vi "Partition_Setup.vi"(8 "error in (no error)":errorcluster, 11 "DataCluster in":T1={"Core"={"Current VI Reference"=refnum, "Close Panel on Exit?"=FALSE, "Exit"=FALSE, "Initialized?"=FALSE}, "Connections"={"cDAQ"={"Task"="ThermTask", "Connected"=FALSE, "Active"=FALSE, "ID"=""}, "Camera"={"Session"="", "Connected"=FALSE, "Active"=FALSE, "Placeholder"=refnum}, "PSU"={"Port"="", "Connected"=FALSE, "Active"=FALSE}, "Arduino"={"Port"="", "Connected"=FALSE, "Active"=FALSE}}, "Data Acquisition"={"Setup"={"Label"="_41", "Operator"="", "Notes"="", "TempGrad"=1.0, "TargetTemp"=-20.0, "Sample Volume"=1.0}, "Camera"={"Image"=refnum, "Save Image"=refnum, "Image Frequency"=20, "Rectangle"={"Left"=0, "Top"=0, "Right"=0, "Bottom"=0, "Rotation"=0.0}, "Calibration"={"Top Left"={"X"=0.0, "Y"=0.0}, "Top Right"={"X"=0.0, "Y"=0.0}, "Bottom Left"={"X"=0.0, "Y"=0.0}, "Bottom Right"={"X"=0.0, "Y"=0.0}, "Fixpoint"={"X"=0.0, "Y"=0.0}, "Scan Area"=0.0, "Fixpoint Area"=0.0, "Well Pixels"=[], "Valid"=FALSE}, "FocusPos"=0, "Display Mapping"=10, "Camera Mode"=10}, "Thermistor"={"Sample Size"=5, "Calibration"={"B0.100"=[3450.0, 3450.0, 3450.0, 3450.0, 3450.0, 3450.0, 3450.0, 3450.0], "R25"=[10.74, 10.74, 10.74, 10.74, 10.74, 10.74, 10.74, 10.74], "c"=[], "State"=[], "V_S"=10.0, "R_S"=10.0}, "Timing Mode"=14713}, "Partition"={"Data"=[], "Cell Label"="", "Cell Color"=0, "Height"=10, "Width"=16, "Grid"=[]}, "Queue"={"Size"=5, "Queue"=refnum}, "Sample Rate"=240, "Active"=FALSE, "Ready"=FALSE, "Graph Mode"=0, "Gradient Buffer"=2}, "Control"={"Sample Rate"=20, "PID gains"={"proportional gain (Kc)"=1.0, "integral time (Ti, min)"=0.01, "derivative time (Td, min)"=0.0}}, "Manual Temp Control"={"TargetTemp"=1.0, "Mode"=0, "Active"=FALSE}} {"Manual Temp Control"."Mode" items=["Cool", "Heat"]; "Manual Temp Control"."TargetTemp" min=-40.0 max=40.0 step=0.5 format="%#_g °C"; "Control"."PID gains"."derivative time (Td, min)" format="%.3f"; "Control"."PID gains"."integral time (Ti, min)" format="%.3f"; "Control"."PID gains"."proportional gain (Kc)" format="%.3f"; "Control"."Sample Rate" min=1 max=20 step=1 format="%.0f Samples/sec"; "Data Acquisition"."Gradient Buffer" min=2 max=30 step=1; "Data Acquisition"."Graph Mode" items=["Thermistor Temperature", "Camera Temperature"]; "Data Acquisition"."Thermistor"."Timing Mode" items=["Automatic"=16097, "High Resolution"=10195, "High Speed"=14712, "Best 50 Hz Rejection"=14713, "Best 60 Hz Rejection"=14714, "Custom"=10137]; "Data Acquisition"."Thermistor"."Calibration"."R_S" min=0.1 max=1000.0 format="%#_g kOhm"; "Data Acquisition"."Thermistor"."Calibration"."V_S" min=5.0 max=48.0 format="%#_g V"; "Data Acquisition"."Thermistor"."Calibration"."R25" min=0.1 max=1000.0 format="%#_g kOhm"; "Data Acquisition"."Thermistor"."Calibration"."B0.100" min=100.0 max=10000.0 format="%#_g K"; "Data Acquisition"."Thermistor"."Sample Size" min=1 max=200; "Data Acquisition"."Sample Rate" min=20 max=240 format="%.0f samples/min"; "Data Acquisition"."Queue"."Size" min=1 max=200; "Data Acquisition"."Camera"."Camera Mode" items=["Temperature Linear", "Signal Linear"]; "Data Acquisition"."Camera"."Display Mapping" items=["Default"=10, "Most Significant Bits"=11, "Full Dynamic"=12, "Downshift"=13, "Given Range"=14, "90% Dynamic"=15, "Given Percent Range"=16]; "Data Acquisition"."Camera"."Calibration"."Fixpoint"."Y" format="%.2f"; "Data Acquisition"."Camera"."Calibration"."Fixpoint"."X" format="%.2f"; "Data Acquisition"."Camera"."Calibration"."Top Left"."Y" format="%.2f"; "Data Acquisition"."Camera"."Calibration"."Top Left"."X" format="%.2f"; "Data Acquisition"."Camera"."Calibration"."Top Right"."Y" format="%.2f"; "Data Acquisition"."Camera"."Calibration"."Top Right"."X" format="%.2f"; "Data Acquisition"."Camera"."Calibration"."Bottom Left"."Y" format="%.2f"; "Data Acquisition"."Camera"."Calibration"."Bottom Left"."X" format="%.2f"; "Data Acquisition"."Camera"."Calibration"."Bottom Right"."Y" format="%.2f"; "Data Acquisition"."Camera"."Calibration"."Bottom Right"."X" format="%.2f"; "Data Acquisition"."Camera"."Rectangle"."Rotation" min=-90.0 max=90.0 step=1.0 format="%.2f"; "Data Acquisition"."Camera"."Rectangle"."Left" scale=0.0..1024.0; "Data Acquisition"."Camera"."Rectangle"."Right" scale=0.0..1024.0; "Data Acquisition"."Camera"."Image Frequency" min=1 max=60 step=1; "Data Acquisition"."Setup"."Sample Volume" min=0.0 max=500.0 format="%#_g µL"; "Data Acquisition"."Setup"."TargetTemp" min=-40.0 max=40.0 step=0.5 format="%#_g °C"; "Data Acquisition"."Setup"."TempGrad" min=-100.0 max=100.0 step=0.1 format="%#_g °C/min"}) -> (0 "error out":errorcluster, 2 "Canceled?":bool, 3 "DataCluster out":T1={"Core"={"Current VI Reference"=refnum, "Close Panel on Exit?"=FALSE, "Exit"=FALSE, "Initialized?"=FALSE}, "Connections"={"cDAQ"={"Task"="ThermTask", "Connected"=FALSE, "Active"=FALSE, "ID"=""}, "Camera"={"Session"="", "Connected"=FALSE, "Active"=FALSE, "Placeholder"=refnum}, "PSU"={"Port"="", "Connected"=FALSE, "Active"=FALSE}, "Arduino"={"Port"="", "Connected"=FALSE, "Active"=FALSE}}, "Data Acquisition"={"Setup"={"Label"="_41", "Operator"="", "Notes"="", "TempGrad"=1.0, "TargetTemp"=-20.0, "Sample Volume"=1.0}, "Camera"={"Image"=refnum, "Save Image"=refnum, "Image Frequency"=20, "Rectangle"={"Left"=0, "Top"=0, "Right"=0, "Bottom"=0, "Rotation"=0.0}, "Calibration"={"Top Left"={"X"=0.0, "Y"=0.0}, "Top Right"={"X"=0.0, "Y"=0.0}, "Bottom Left"={"X"=0.0, "Y"=0.0}, "Bottom Right"={"X"=0.0, "Y"=0.0}, "Fixpoint"={"X"=0.0, "Y"=0.0}, "Scan Area"=0.0, "Fixpoint Area"=0.0, "Well Pixels"=[], "Valid"=FALSE}, "FocusPos"=0, "Display Mapping"=10, "Camera Mode"=10}, "Thermistor"={"Sample Size"=5, "Calibration"={"B0.100"=[3450.0, 3450.0, 3450.0, 3450.0, 3450.0, 3450.0, 3450.0, 3450.0], "R25"=[10.74, 10.74, 10.74, 10.74, 10.74, 10.74, 10.74, 10.74], "c"=[], "State"=[], "V_S"=10.0, "R_S"=10.0}, "Timing Mode"=14713}, "Partition"={"Data"=[["A", "20%", "", "", ""], ["B", "30", "", "", ""], ["C", "5%", "", "", ""], ["D", "35%", "", "", ""], ["E", "...", "", "", ""], ["F", "...", "", "", ""], ["G", "...", "", "", ""], ["X", "Empty", "", "", ""]], "Cell Label"="A", "Cell Color"=29373, "Height"=8, "Width"=12, "Grid"=[["X", "X", "X", "X", "X", "X", "X", "X", "X", "X", "X", "X"], ["X", "X", "X", "X", "X", "X", "X", "X", "X", "X", "X", "X"], ["X", "X", "X", "X", "X", "X", "X", "X", "X", "X", "X", "X"], ["X", "X", "X", "X", "X", "X", "X", "X", "X", "X", "X", "X"], ["X", "X", "X", "X", "X", "X", "X", "X", "X", "X", "X", "X"], ["X", "X", "X", "X", "X", "X", "X", "X", "X", "X", "X", "X"], ["X", "X", "X", "X", "X", "X", "X", "X", "X", "X", "X", "X"], ["X", "X", "X", "X", "X", "X", "X", "X", "X", "X", "X", "X"]]}, "Queue"={"Size"=5, "Queue"=refnum}, "Sample Rate"=240, "Active"=FALSE, "Ready"=FALSE, "Graph Mode"=0, "Gradient Buffer"=2}, "Control"={"Sample Rate"=20, "PID gains"={"proportional gain (Kc)"=1.0, "integral time (Ti, min)"=0.01, "derivative time (Td, min)"=0.0}}, "Manual Temp Control"={"TargetTemp"=1.0, "Mode"=0, "Active"=FALSE}} {"Manual Temp Control"."Mode" items=["Cool", "Heat"]; "Manual Temp Control"."TargetTemp" min=-40.0 max=40.0 step=0.5 format="%#_g °C"; "Control"."PID gains"."derivative time (Td, min)" format="%.3f"; "Control"."PID gains"."integral time (Ti, min)" format="%.3f"; "Control"."PID gains"."proportional gain (Kc)" format="%.3f"; "Control"."Sample Rate" min=1 max=20 step=1 format="%.0f Samples/sec"; "Data Acquisition"."Gradient Buffer" min=2 max=30 step=1; "Data Acquisition"."Graph Mode" items=["Thermistor Temperature", "Camera Temperature"]; "Data Acquisition"."Thermistor"."Timing Mode" items=["Automatic"=16097, "High Resolution"=10195, "High Speed"=14712, "Best 50 Hz Rejection"=14713, "Best 60 Hz Rejection"=14714, "Custom"=10137]; "Data Acquisition"."Thermistor"."Calibration"."R_S" min=0.1 max=1000.0 format="%#_g kOhm"; "Data Acquisition"."Thermistor"."Calibration"."V_S" min=5.0 max=48.0 format="%#_g V"; "Data Acquisition"."Thermistor"."Calibration"."R25" min=0.1 max=1000.0 format="%#_g kOhm"; "Data Acquisition"."Thermistor"."Calibration"."B0.100" min=100.0 max=10000.0 format="%#_g K"; "Data Acquisition"."Thermistor"."Sample Size" min=1 max=200; "Data Acquisition"."Sample Rate" min=20 max=240 format="%.0f samples/min"; "Data Acquisition"."Queue"."Size" min=1 max=200; "Data Acquisition"."Camera"."Camera Mode" items=["Temperature Linear", "Signal Linear"]; "Data Acquisition"."Camera"."Display Mapping" items=["Default"=10, "Most Significant Bits"=11, "Full Dynamic"=12, "Downshift"=13, "Given Range"=14, "90% Dynamic"=15, "Given Percent Range"=16]; "Data Acquisition"."Camera"."Calibration"."Fixpoint"."Y" format="%.2f"; "Data Acquisition"."Camera"."Calibration"."Fixpoint"."X" format="%.2f"; "Data Acquisition"."Camera"."Calibration"."Top Left"."Y" format="%.2f"; "Data Acquisition"."Camera"."Calibration"."Top Left"."X" format="%.2f"; "Data Acquisition"."Camera"."Calibration"."Top Right"."Y" format="%.2f"; "Data Acquisition"."Camera"."Calibration"."Top Right"."X" format="%.2f"; "Data Acquisition"."Camera"."Calibration"."Bottom Left"."Y" format="%.2f"; "Data Acquisition"."Camera"."Calibration"."Bottom Left"."X" format="%.2f"; "Data Acquisition"."Camera"."Calibration"."Bottom Right"."Y" format="%.2f"; "Data Acquisition"."Camera"."Calibration"."Bottom Right"."X" format="%.2f"; "Data Acquisition"."Camera"."Rectangle"."Rotation" min=-90.0 max=90.0 step=1.0 format="%.2f"; "Data Acquisition"."Camera"."Rectangle"."Left" scale=0.0..1024.0; "Data Acquisition"."Camera"."Rectangle"."Right" scale=0.0..1024.0; "Data Acquisition"."Camera"."Image Frequency" min=1 max=60 step=1; "Data Acquisition"."Setup"."Sample Volume" min=0.0 max=500.0 format="%#_g µL"; "Data Acquisition"."Setup"."TargetTemp" min=-40.0 max=40.0 step=0.5 format="%#_g °C"; "Data Acquisition"."Setup"."TempGrad" min=-100.0 max=100.0 step=0.1 format="%#_g °C/min"})   [LabVIEW 2024]
uses:
  DataCluster.ctl
  <vilib>/userDefined/High Color/IMAQdx.ctl
  <vilib>/vision/Image Controls.llb/IMAQ Image.ctl
  <vilib>/Utility/miscctls.llb/LVRowAndColumnTypeDef.ctl
  <vilib>/Utility/miscctls.llb/LVBoundsTypeDef.ctl
  <vilib>/Utility/xml.llb/Write to XML File(string).vi
  <vilib>/Utility/xml.llb/Read From XML File(string).vi
panel:
  out "Grid":string[][](table)=[["X", "X", "X", "X", "X", "X", "X", "X", "X", "X", "X", "X"], ["X", "X", "X", "X", "X", "X", "X", "X", "X", "X", "X", "X"], ["X", "X", "X", "X", "X", "X", "X", "X", "X", "X", "X", "X"], ["X", "X", "X", "X", "X", "X", "X", "X", "X", "X", "X", "X"], ["X", "X", "X", "X", "X", "X", "X", "X", "X", "X", "X", "X"], ["X", "X", "X", "X", "X", "X", "X", "X", "X", "X", "X", "X"], ["X", "X", "X", "X", "X", "X", "X", "X", "X", "X", "X", "X"], ["X", "X", "X", "X", "X", "X", "X", "X", "X", "X", "X", "X"]]
  in  "Cancel":bool
  in  "OK":bool
  in  "Partition Size":enum32{"12x8", "24x16"}(radio)
  in  "Partitions":i32[](listbox)=[0]
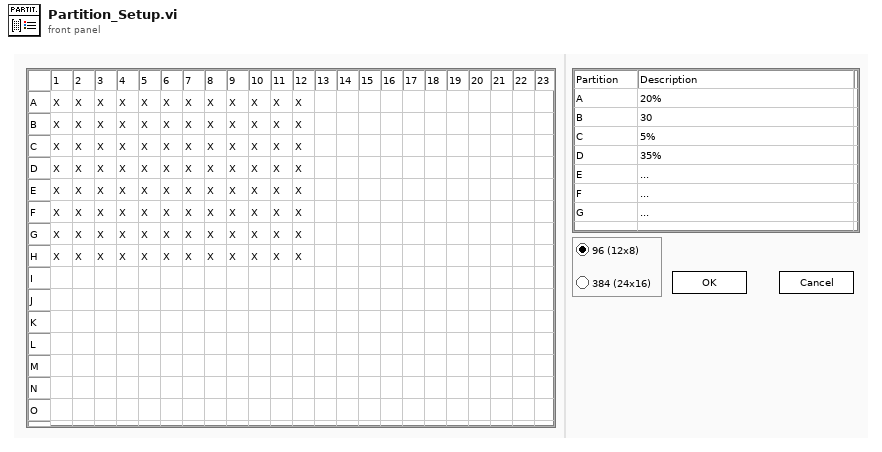
[diagram p1: front panel]
types:
  T1 = typedef "DataCluster.ctl" = cluster{"Core":cluster{"Current VI Reference":refnum<vi>, "Close Panel on Exit?":bool, "Exit":bool, "Initialized?":bool}, "Connections":cluster{"cDAQ":cluster{"Task":refnum<k21>, "Connected":bool, "Active":bool, "ID":string}, "Camera":cluster{"Session":T2, "Connected":bool, "Active":bool, "Placeholder":T3}, "PSU":cluster{"Port":refnum<visa-resource-name>, "Connected":bool, "Active":bool}, "Arduino":cluster{"Port":refnum<visa-resource-name>, "Connected":bool, "Active":bool}}, "Data Acquisition":cluster{"Setup":cluster{"Label":string, "Operator":string, "Notes":string, "TempGrad":dbl, "TargetTemp":dbl, "Sample Volume":dbl}, "Camera":cluster{"Image":T3, "Save Image":T3, "Image Frequency":i32, "Rectangle":T4, "Calibration":cluster{"Top Left":T5, "Top Right":T5, "Bottom Left":T5, "Bottom Right":T5, "Fixpoint":T5, "Scan Area":dbl, "Fixpoint Area":dbl, "Well Pixels":cluster{"X":i32, "Y":i32}[][], "Valid":bool}, "FocusPos":u32, "Display Mapping":u32, "Camera Mode":u32}, "Thermistor":cluster{"Sample Size":i32, "Calibration":cluster{"B0.100":dbl[], "R25":dbl[], "c":dbl[][], "State":bool[], "V_S":dbl, "R_S":dbl}, "Timing Mode":i32}, "Partition":cluster{"Data":string[][], "Cell Label":string, "Cell Color":u32, "Height":i32, "Width":i32, "Grid":string[][]}, "Queue":cluster{"Size":i32, "Queue":refnum<queue>}, "Sample Rate":i32, "Active":bool, "Ready":bool, "Graph Mode":u16, "Gradient Buffer":i32}, "Control":cluster{"Sample Rate":i32, "PID gains":cluster{"proportional gain (Kc)":dbl, "integral time (Ti, min)":dbl, "derivative time (Td, min)":dbl}}, "Manual Temp Control":cluster{"TargetTemp":dbl, "Mode":u16, "Active":bool}}
  T2 = typedef "IMAQdx.ctl" = refnum<k21>
  T3 = typedef "IMAQ Image.ctl" = refnum<image>
  T4 = typedef "IMAQ Rectangle" = cluster{"Left":i32, "Top":i32, "Right":i32, "Bottom":i32, "Rotation":dbl}
  T5 = typedef "IMAQ Point" = cluster{"X":sgl, "Y":sgl}
  T6 = typedef "LVRowAndColumnTypeDef.ctl" = cluster{"Row":i32, "Column":i32}
  T7 = cluster{"Data":string[][], "Cell Label":string, "Cell Color":u32, "Height":i32, "Width":i32, "Grid":string[][]}
  T8 = typedef "LVBoundsTypeDef.ctl" = cluster{"Width":u32, "Height":u32}
  T9 = typedef "LVRectTypeDef.ctl" = cluster{"Left":i16, "Top":i16, "Right":i16, "Bottom":i16}
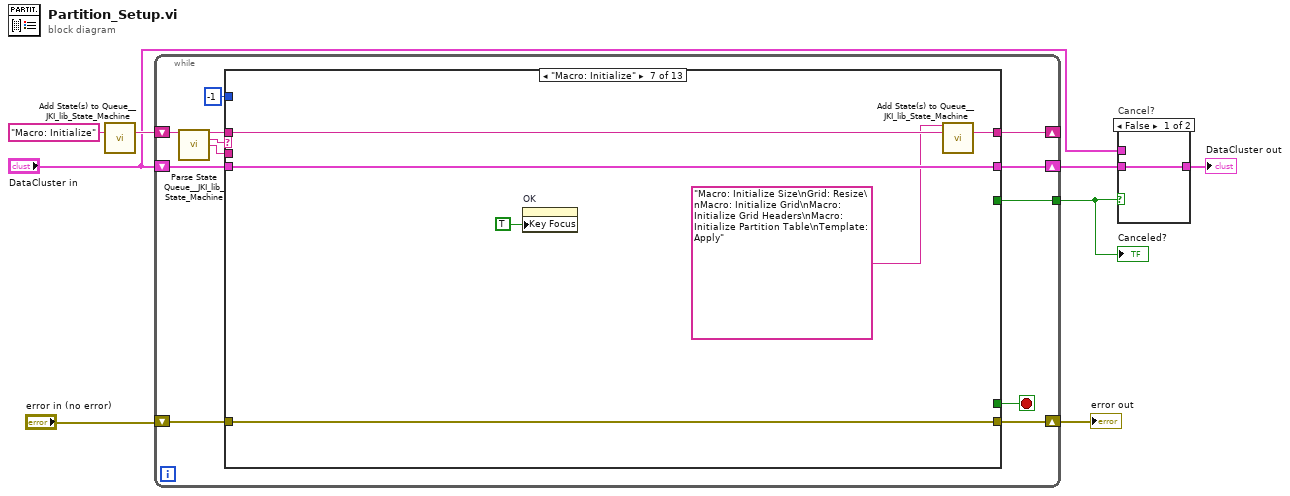
[diagram p0: block diagram]
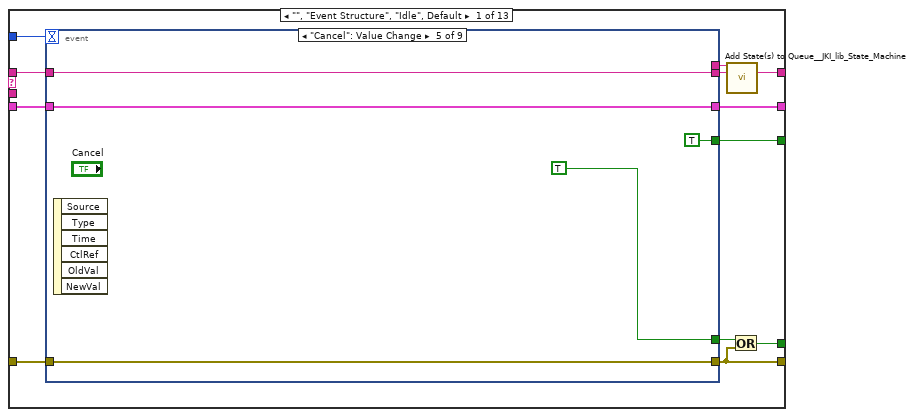
[diagram p3: hidden frame]
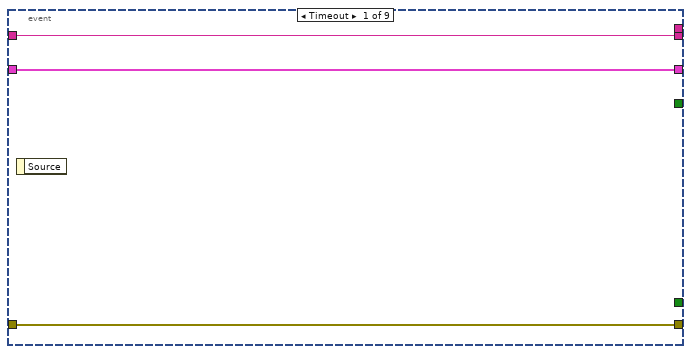
[diagram p4: hidden frame]
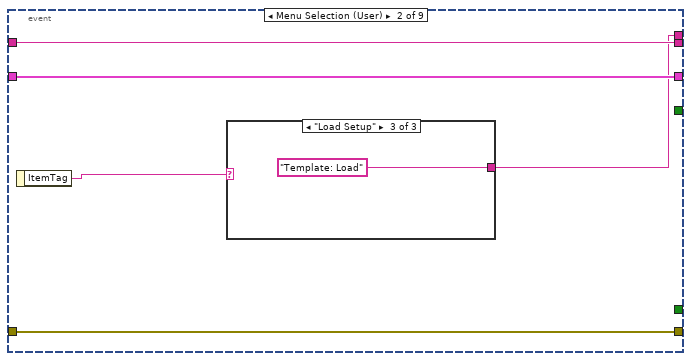
[diagram p5: hidden frame]
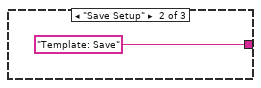
[diagram p7: hidden frame]
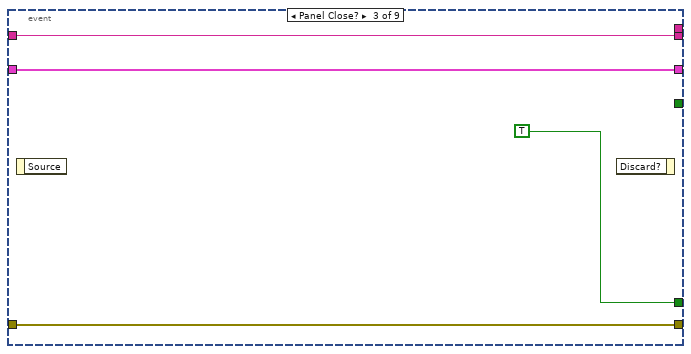
[diagram p8: hidden frame]
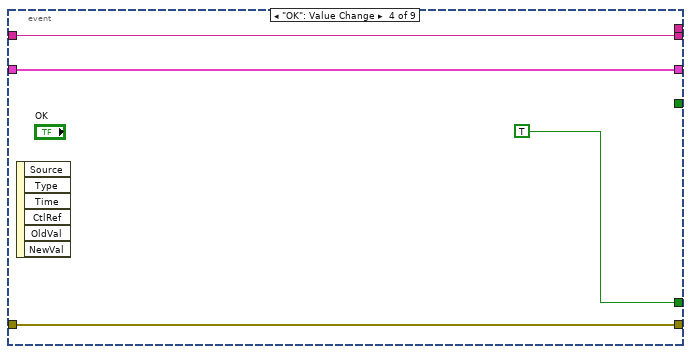
[diagram p9: hidden frame]
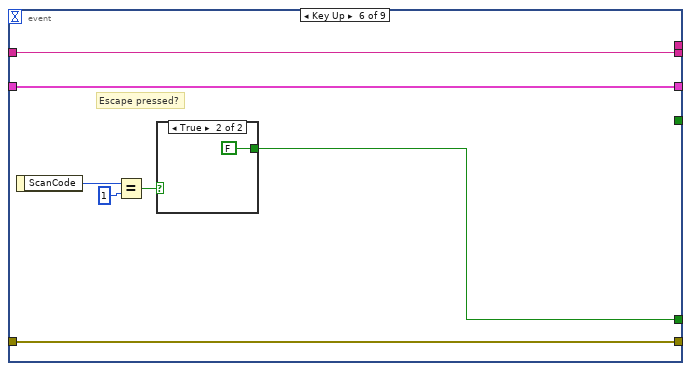
[diagram p10: hidden frame]
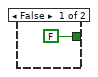
[diagram p11: hidden frame]
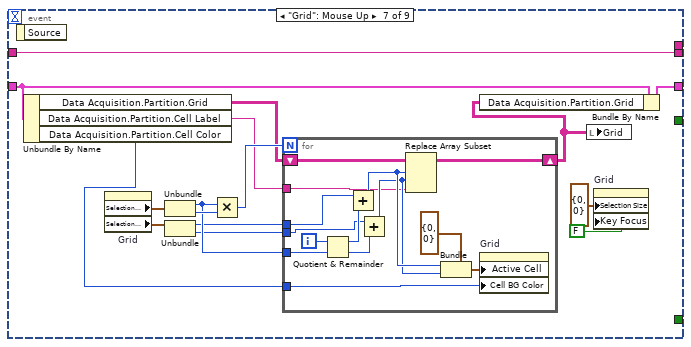
[diagram p12: hidden frame]
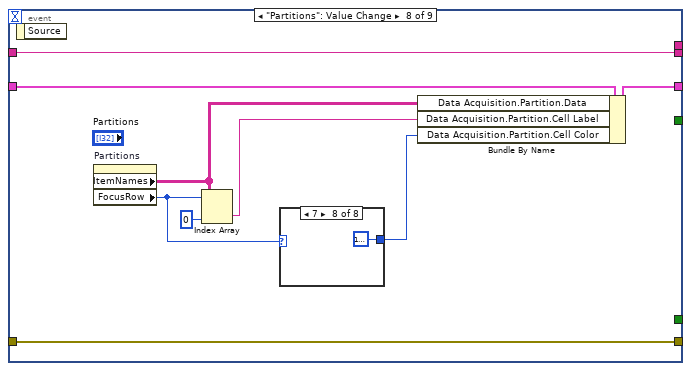
[diagram p13: hidden frame]
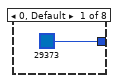
[diagram p14: hidden frame]
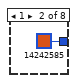
[diagram p15: hidden frame]
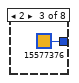
[diagram p16: hidden frame]
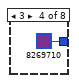
[diagram p17: hidden frame]
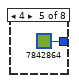
[diagram p18: hidden frame]
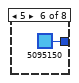
[diagram p19: hidden frame]
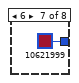
[diagram p20: hidden frame]
diagram:
  n1 = call <vilib>:"Add State(s) to Queue__JKI_lib_State_Machine.vi"("State(s) in (\"\")"="Macro: Initialize") -> ("States Out"=w5:string)  [unwired: 14 in]
  n2 = while {
    shift-right: [w20] -> w3
    shift-left: "DataCluster in" -> [w19]
    shift-right: [w15] -> w8
    shift-left: "error in (no error)" -> [w16]
    shift-right: [w10] -> _
    shift-left: w5 -> [w14]
    tunnel: [w9] -> w2
    stop <- w17 stop-if-true
    n3 = call <vilib>:"Parse State Queue__JKI_lib_State_Machine.vi"("State Queue"=w14) -> ("Remaining States"=w11:string, "Current State"=w13:string, "Arguments"=w12:string)  [unwired: 12 in]
    n4 = case shown="\"Macro: Initialize\"" w13 {
      tunnel: [w32 w126 w143 w158 w187 w215 w221 w229 w246 w250 w265 w295 w327] -> w20
      tunnel: w19 -> [w31 w126 w143 w157 w187 w215 w221 w225 w246 w250 w265 w299 w327]
      tunnel: -1 -> [w29 _ _ _ _ _ _ _ _ _ _ _ _]
      tunnel: [w28 _ _ _ _ _ _ _ _ _ _ _ _] -> w17
      tunnel: w16 -> [w27 w127 w147 w175 w193 w216 w222 w232 w249 w255 w268 w303 w336]
      tunnel: [w26 w127 w147 w175 w193 w216 w222 w232 w249 w255 w268 w303 w336] -> w15
      tunnel: w12 -> [_ _ _ _ _ _ _ _ _ _ _ _ _]
      tunnel: w11 -> [w25 w124 w145 w173 w191 w213 w219 w230 w247 w253 w266 w301 w334]
      tunnel: [w23 w125 w146 w174 w192 w214 w220 w231 w248 w254 w267 w302 w335] -> w10
      tunnel: [w21 _ _ _ _ _ _ _ _ _ _ _ _] -> w9
      frame "", "Event Structure", "Idle", Default {
        n5 = event shown="[4] \"Cancel\": Value Change" {
          selector: _ -> [_ _ _ _ _ _ _ _ _]
          dyn-events: _ -> [_ _ _ _ _ _ _ _ _]
          timeout: w29 -> [_ _ _ _ _ _ _ _ _]
          tunnel: w31 -> [w33 w39 w44 w48 w53 w57 w71 w103 w119]
          tunnel: [w33 w39 w44 w48 w53 w57 w68 w100 w118] -> w32
          tunnel: [_ _ TRUE TRUE TRUE w62 _ _ _] -> w30
          tunnel: [w35 w40 w45 w49 w54 w58 _ w98 w116] -> w26
          tunnel: w27 -> [w35 w40 w45 w49 w54 w58 _ w98 w116]
          tunnel: [w34 w38 w43 w47 w52 w56 w72 w99 w117] -> w24
          tunnel: w25 -> [w34 w38 w43 w47 w52 w56 w72 w99 w117]
          tunnel: [_ w37 _ _ _ _ _ _ "Macro: Initialize Grid\nGrid: Resize\nMacro: Initialize Grid Headers\nMacro: Empty Grid" ("State(s) in Front (\"\")")] -> w22
          tunnel: [_ _ _ _ TRUE _ _ _ _] -> w21
          event Timeout {
            n6 = event-data() -> ()  [unwired: 1 in, 1 out]
          }
          event Menu Selection (User) {
            n7 = event-data() -> ("ItemTag"=w36:string)  [unwired: 1 in]
            n8 = case shown="\"Load Setup\"" w36 {
              tunnel: [_ "Template: Save" "Template: Load"] -> w37
              frame "False", Default {
              }
              frame "Save Setup" {
              }
              frame "Load Setup" {
              }
            }
          }
          event Panel Close? {
            n9 = event-data() -> ()  [unwired: 1 in, 1 out]
            n10 = event-data() -> ()  [unwired: 2 in, 1 out]
          }
          event "OK": Value Change {
            n11 = event-data() -> ()  [unwired: 1 in, 6 out]
          }
          event "Cancel": Value Change {
            n12 = event-data() -> ()  [unwired: 1 in, 6 out]
          }
          event Key Up {
            # "Escape pressed?"
            n13 = event-data() -> ("ScanCode"=w61:i16)  [unwired: 1 in]
            n14 = Equal?(x=w61, y=i16 1) -> (x = y?=w59:bool)
            n15 = case shown="True" w59 {
              tunnel: [FALSE FALSE] -> w62
              frame False {
              }
              frame True {
              }
            }
          }
          event "Grid": Mouse Up {
            n16 = event-data() -> ()  [unwired: 1 in, 1 out]
            n17 = Unbundle By Name(w71) -> ("Data Acquisition.Partition.Grid"=w66:string[][], "Data Acquisition.Partition.Cell Label"=w70:string, "Data Acquisition.Partition.Cell Color"=w69:u32)
            n18 = property on="Grid" class="Tbl (strict)"() -> ("Selection Size"=w79:T6, "Selection Start"=w76:T6)  [unwired: 2 in, 2 out]
            n19 = Unbundle(w79) -> ("Row"=w77:i32, "Column"=w78:i32)
            n20 = Unbundle(w76) -> ("Row"=w75:i32, "Column"=w74:i32)
            n21 = Multiply(x=w77, y=w78) -> (x*y=w80:i32)
            n22 = for {
              N: w80 -> [_]
              tunnel: w77 -> [w94]
              shift-right: [w90] -> w67
              shift-left: w66 -> [w81]
              tunnel: w75 -> [w89]
              tunnel: w74 -> [w88]
              tunnel: w70 -> [w83]
              tunnel: w69 -> [w82]
              i -> [w93]
              n23 = Quotient & Remainder(x=w93, y=w94) -> (x-y*floor(x/y)=w92:i32, floor(x/y)=w91:i32)
              n24 = Add(x=w89, y=w92) -> (x+y=w85:i32)
              n25 = Add(x=w88, y=w91) -> (x+y=w84:i32)
              n26 = Replace Array Subset(array=w81, new element=w83, index (row)=w85, index (col)=w84) -> (w90:string[][])
              n27 = Bundle(cluster=T6 {"Row"=0, "Column"=0} ("Active Cell:Active Cell"), "Row"=w85, "Column"=w84) -> (w86:T6)
              n28 = property on="Grid" class="Tbl (strict)"("Active Cell"=w86, "Cell BG Color"=w82) -> ()  [unwired: 2 in, 2 out]
            }
            n29 = Bundle By Name(cluster=w71, "Data Acquisition.Partition.Grid"=w67) -> (w68:T1)
            n30 = local write "Grid"(w67) -> ()
            n31 = property on="Grid" class="Tbl (strict)"("Selection Size"=T6 {"Row"=0, "Column"=0} ("Selection Start"), "Key Focus"=FALSE) -> ()  [unwired: 2 in, 2 out]
          }
          event "Partitions": Value Change {
            n32 = event-data() -> ()  [unwired: 1 in, 1 out]
            n33 = property on="Partitions" class="MCListbox (strict)"() -> ("ItemNames"=w95:string[][], "FocusRow"=w101:i32)  [unwired: 2 in, 2 out]
            n34 = Index Array(array=w95, index (row)=w101, index (col)=0 ("disabled index (col)")) -> (element=w97:string)
            n35 = case shown="7" w101 {
              tunnel: [u32 29373 ("Active Cell:Cell Background Color") u32 14242585 ("Active Cell:Cell Background Color") u32 15577376 ("Active Cell:Cell Background Color") u32 8269710 ("Active Cell:Cell Background Color") u32 7842864 ("Active Cell:Cell Background Color") u32 5095150 ("Active Cell:Cell Background Color") u32 10621999 ("Active Cell:Cell Background Color") u32 16777216 ("Active Cell:Cell Background Color")] -> w96
              frame 0, Default {
              }
              frame 1 {
              }
              frame 2 {
              }
              frame 3 {
              }
              frame 4 {
              }
              frame 5 {
              }
              frame 6 {
              }
              frame 7 {
              }
            }
            n36 = Bundle By Name(cluster=w103, "Data Acquisition.Partition.Data"=w95, "Data Acquisition.Partition.Cell Label"=w97, "Data Acquisition.Partition.Cell Color"=w96) -> (w100:T1)
          }
          event "Partition Size": Value Change {
            n37 = event-data() -> ()  [unwired: 1 in, 1 out]
            n38 = case shown="\"12x8\", Default" "Partition Size" {
              tunnel: [8 ("Data Acquisition.Partition.Height") 16 ("Data Acquisition.Partition.Height")] -> w114
              tunnel: [12 ("Data Acquisition.Partition.Width") 24 ("Data Acquisition.Partition.Width")] -> w113
              frame "12x8", Default {
              }
              frame "24x16" {
              }
            }
            n39 = Bundle By Name(cluster=w119, "Data Acquisition.Partition.Height"=w114, "Data Acquisition.Partition.Width"=w113) -> (w118:T1)
          }
        }
        n40 = call <vilib>:"Add State(s) to Queue__JKI_lib_State_Machine.vi"("State(s) in Front (\"\")"=w22, "State(s) in (\"\")"=w24) -> ("States Out"=w23:string)  [unwired: 13 in]
        n41 = Or(x=w30, y=w26) -> (x .or. y?=w28:bool)
      }
      frame "---------- Template ----------" {
        n42 = call <vilib>:"Add State(s) to Queue__JKI_lib_State_Machine.vi"("State(s) in (\"\")"=w124) -> ("States Out"=w125:string)  [unwired: 14 in]
      }
      frame "Template: Save" {
        n43 = call <vilib>:"Application Directory.vi"() -> ("Application Directory"=w139:path)
        n44 = Build Path(base path=w139, name or relative path=path "Partitions") -> (appended path=w140:path)
        n45 = call <vilib>:"Check if File or Folder Exists.vi"("path"=w140) -> ("file or folder exists?"=w142:bool, "dup path"=w141:path)  [unwired: 8 in, 1 out]
        n46 = case shown="False" w142 {
          tunnel: w141 -> [w149 w150]
          tunnel: [w148 w150] -> w133
          frame False {
            n47 = Create Folder(path (use dialog)=w149) -> (created path=w148:path)  [unwired: 2 in, 2 out]
          }
          frame True {
          }
        }
        n48 = Unbundle By Name(w143) -> ("Data Acquisition.Partition"=w144:T7)
        n49 = call "File Dialog3"("start path"=w133, "prompt"="Save Parition Tempalte", "button label"="Save Template", "default name"="Partition Setup", "pattern (all files)"="*.prt", "pattern label"="Partition Template") -> ("selected path"=w136:path, "cancelled"=w134:bool, "error out"=w135:errorcluster)  [unwired: 6 in, 1 out]
        n50 = Or(x=w134, y=w135) -> (x .or. y?=w137:bool)
        n51 = case shown="False" w137 {
          tunnel: w144 -> [w153 _]
          tunnel: w136 -> [w151 _]
          frame False {
            n52 = Flatten To XML(6:w153) -> (2:w152:string)
            n53 = call-poly <vilib>:"Write to XML File.vi"("XML Input"=w152, "XML File Path"=w151) -> ()  [unwired: 7 in, 3 out]
          }
          frame True {
          }
        }
        n54 = call <vilib>:"Add State(s) to Queue__JKI_lib_State_Machine.vi"("State(s) in (\"\")"=w145) -> ("States Out"=w146:string)  [unwired: 14 in]
      }
      frame "Template: Load" {
        n55 = call <vilib>:"Application Directory.vi"() -> ("Application Directory"=w167:path)
        n56 = Build Path(base path=w167, name or relative path=path "Partitions") -> (appended path=w168:path)
        n57 = call <vilib>:"Check if File or Folder Exists.vi"("path"=w168) -> ("file or folder exists?"=w170:bool, "dup path"=w169:path)  [unwired: 8 in, 1 out]
        n58 = case shown="False" w170 {
          tunnel: w169 -> [w177 w178]
          tunnel: [w176 w178] -> w171
          frame False {
            n59 = Create Folder(path (use dialog)=w177) -> (created path=w176:path)  [unwired: 2 in, 2 out]
          }
          frame True {
          }
        }
        n60 = Unbundle By Name(w157) -> ("Data Acquisition.Partition"=w172:T7)
        n61 = call "File Dialog2"("start path"=w171, "prompt"="Load Parition Tempalte", "button label"="Load Template", "default name"="Partition Setup", "pattern (all files)"="*.prt", "pattern label"="Partition Template") -> ("selected path"=w160:path, "cancelled"=w159:bool)  [unwired: 6 in, 2 out]
        n62 = case shown="False" w159 {
          tunnel: w172 -> [w181 w183]
          tunnel: w160 -> [w182 _]
          tunnel: [w179 w183] -> w155
          frame False {
            n63 = call-poly <vilib>:"Read From XML File.vi"("XML File Path"=w182) -> ("XML Elements"=w180:string)  [unwired: 8 in, 2 out]
            n64 = Unflatten From XML(xml string=w180, type=w181) -> (value=w179:T7)  [unwired: 1 in, 1 out]
          }
          frame True {
          }
        }
        n65 = Bundle By Name(cluster=w157, "Data Acquisition.Partition"=w155) -> (w158:T1)
        n66 = Unbundle By Name(w155) -> ("Grid"=w154:string[][])
        n67 = local write "Grid"(w154) -> ()
        n68 = call <vilib>:"Add State(s) to Queue__JKI_lib_State_Machine.vi"("State(s) in Front (\"\")"="Grid: Resize\nMacro: Initialize Grid Headers\nTemplate: Apply" ("State(s) in Front (\"\")"), "State(s) in (\"\")"=w173) -> ("States Out"=w174:string)  [unwired: 13 in]
      }
      frame "Template: Apply" {
        n69 = Unbundle By Name(w187) -> ("Data Acquisition.Partition.Grid"=w186:string[][], "Data Acquisition.Partition.Data"=w190:string[][], "Data Acquisition.Partition.Height"=w188:i32, "Data Acquisition.Partition.Width"=w185:i32)
        n70 = case shown="12, Default" w185 {
          tunnel: [1 0] -> w184
          frame 24 {
          }
          frame 12, Default {
          }
        }
        n71 = local write "Partition Size"(w184) -> ()
        n72 = Multiply(x=w188, y=w185) -> (x*y=w189:i32)
        n73 = for {
          N: w189 -> [_]
          tunnel: w188 -> [w204]
          tunnel: w186 -> [w200]
          i -> [w203]
          n74 = Quotient & Remainder(x=w203, y=w204) -> (x-y*floor(x/y)=w199:i32, floor(x/y)=w198:i32)
          n75 = Index Array(array=w200, index (row)=w199, index (col)=w198) -> (element=w197:string)
          n76 = case shown="\"X\"" w197 {
            tunnel: [u32 29373 ("Active Cell:Cell Background Color") u32 14242585 ("Active Cell:Cell Background Color") u32 15577376 ("Active Cell:Cell Background Color") u32 8269710 ("Active Cell:Cell Background Color") u32 7842864 ("Active Cell:Cell Background Color") u32 5095150 ("Active Cell:Cell Background Color") u32 10621999 ("Active Cell:Cell Background Color") u32 16777216 ("Active Cell:Cell Background Color")] -> w196
            frame "A", Default {
            }
            frame "B" {
            }
            frame "C" {
            }
            frame "D" {
            }
            frame "E" {
            }
            frame "F" {
            }
            frame "G" {
            }
            frame "X" {
            }
          }
          n77 = Bundle(cluster=T6 {"Row"=0, "Column"=0} ("Active Cell:Active Cell"), "Row"=w199, "Column"=w198) -> (w201:T6)
          n78 = property on="Grid" class="Tbl (strict)"("Active Cell"=w201, "Cell BG Color"=w196) -> ()  [unwired: 2 in, 2 out]
        }
        n79 = property on="Partitions" class="MCListbox (strict)"("ItemNames"=w190) -> ()  [unwired: 2 in, 2 out]
        n80 = call <vilib>:"Add State(s) to Queue__JKI_lib_State_Machine.vi"("State(s) in (\"\")"=w191) -> ("States Out"=w192:string)  [unwired: 14 in]
      }
      frame "---------- Macro ----------" {
        n81 = call <vilib>:"Add State(s) to Queue__JKI_lib_State_Machine.vi"("State(s) in (\"\")"=w213) -> ("States Out"=w214:string)  [unwired: 14 in]
      }
      frame "Macro: Initialize" {
        n82 = property on="OK" class="Bool"("Key Focus"=TRUE) -> ()  [unwired: 2 in, 2 out]
        n83 = call <vilib>:"Add State(s) to Queue__JKI_lib_State_Machine.vi"("State(s) in Front (\"\")"="Macro: Initialize Size\nGrid: Resize\nMacro: Initialize Grid\nMacro: Initialize Grid Headers\nMacro: Initialize Partition Table\nTemplate: Apply" ("State(s) in Front (\"\")"), "State(s) in (\"\")"=w219) -> ("States Out"=w220:string)  [unwired: 13 in]
      }
      frame "Macro: Initialize Partition Table" {
        w223 = T6 {"Row"=0, "Column"=0} ("Selected Cell")
        n84 = for {
          N: 8 -> [_]
          i -> [w234]
          n85 = Bundle(w234, 0) -> (w235:cluster{i32, i32})  [unwired: 1 in]
          n86 = case shown="7" w234 {
            tunnel: [u32 29373 ("Active Cell:Cell Background Color") u32 14242585 ("Active Cell:Cell Background Color") u32 15577376 ("Active Cell:Cell Background Color") u32 8269710 ("Active Cell:Cell Background Color") u32 7842864 ("Active Cell:Cell Background Color") u32 5095150 ("Active Cell:Cell Background Color") u32 10621999 ("Active Cell:Cell Background Color") u32 16777216 ("Active Cell:Cell Background Color")] -> w233
            frame 0, Default {
            }
            frame 1 {
            }
            frame 2 {
            }
            frame 3 {
            }
            frame 4 {
            }
            frame 5 {
            }
            frame 6 {
            }
            frame 7 {
            }
          }
          n87 = property on="Partitions" class="MCListbox (strict)"("ActiveCell"=w235, "CellBG"=w233) -> ()  [unwired: 2 in, 2 out]
        }
        n88 = property on="Partitions" class="MCListbox (strict)"() -> ("ItemNames"=w228:string[][])  [unwired: 2 in, 2 out]
        n89 = Bundle By Name(cluster=w225, "Data Acquisition.Partition.Data"=w228, "Data Acquisition.Partition.Cell Label"="A", "Data Acquisition.Partition.Cell Color"=u32 29373 ("Active Cell:Cell Background Color")) -> (w229:T1)
        n90 = property on="Partitions" class="MCListbox (strict)"("SelectedCell"=w223, "TopLeft"=w223) -> ()  [unwired: 2 in, 2 out]
        n91 = call <vilib>:"Add State(s) to Queue__JKI_lib_State_Machine.vi"("State(s) in (\"\")"=w230) -> ("States Out"=w231:string)  [unwired: 14 in]
      }
      frame "Macro: Initialize Grid" {
        n92 = Unbundle By Name(w246) -> ("Data Acquisition.Partition.Grid"=→"Grid":string[][])
        n93 = call <vilib>:"Add State(s) to Queue__JKI_lib_State_Machine.vi"("State(s) in (\"\")"=w247) -> ("States Out"=w248:string)  [unwired: 14 in]
      }
      frame "Macro: Initialize Size" {
        n94 = Unbundle By Name(w250) -> ("Data Acquisition.Partition.Width"=w251:i32)
        n95 = case shown="12, Default" w251 {
          tunnel: [1 0] -> w252
          frame 24 {
          }
          frame 12, Default {
          }
        }
        n96 = local write "Partition Size"(w252) -> ()
        n97 = call <vilib>:"Add State(s) to Queue__JKI_lib_State_Machine.vi"("State(s) in (\"\")"=w253) -> ("States Out"=w254:string)  [unwired: 14 in]
      }
      frame "Macro: Initialize Grid Headers" {
        n98 = Unbundle By Name(w265) -> ("Data Acquisition.Partition.Width"=w260:i32, "Data Acquisition.Partition.Height"=w259:i32)
        n99 = for {
          N: w260 -> [_]
          shift-right: [w292] -> w263
          shift-left: string[] [] -> [w290]
          i -> [w293]
          n100 = Increment(x=w293) -> (x+1=w289:i32)
          n101 = Number To Decimal String(number=w289) -> (decimal integer string=w291:string)  [unwired: 1 in]
          n102 = Build Array (concatenate)(w290, w291) -> (w292:string[])
        }
        n103 = for {
          N: w259 -> [_]
          shift-right: [w270] -> w264
          shift-left: string[] [] -> [w269]
          i -> [w272]
          n104 = case shown="15" w272 {
            tunnel: ["A" "B" "C" "D" "E" "F" "G" "H" "I" "J" "K" "L" "M" "N" "O" "P"] -> w271
            frame 0, Default {
            }
            frame 1 {
            }
            frame 2 {
            }
            frame 3 {
            }
            frame 4 {
            }
            frame 5 {
            }
            frame 6 {
            }
            frame 7 {
            }
            frame 8 {
            }
            frame 9 {
            }
            frame 10 {
            }
            frame 11 {
            }
            frame 12 {
            }
            frame 13 {
            }
            frame 14 {
            }
            frame 15 {
            }
          }
          n105 = Build Array (concatenate)(w269, w271) -> (w270:string[])
        }
        n106 = property on="Grid" class="Tbl (strict)"("Column Headers[]"=w263, "Row Headers[]"=w264) -> ()  [unwired: 2 in, 2 out]
        n107 = Wait (ms)(milliseconds to wait=u32 20) -> ()  [unwired: 1 out]
        n108 = call <vilib>:"Add State(s) to Queue__JKI_lib_State_Machine.vi"("State(s) in (\"\")"=w266) -> ("States Out"=w267:string)  [unwired: 14 in]
      }
      frame "Macro: Empty Grid" {
        n109 = Unbundle By Name(w299) -> ("Data Acquisition.Partition.Height"=w297:i32, "Data Acquisition.Partition.Width"=w296:i32)
        n110 = Multiply(x=w297, y=w296) -> (x*y=w300:i32)
        n111 = for {
          N: w300 -> [_]
          tunnel: w296 -> [w309]
          i -> [w310]
          (unwired) T8 {"Width"=20, "Height"=20} ("Size")
          n112 = Quotient & Remainder(x=w310, y=w309) -> (x-y*floor(x/y)=w304:i32, floor(x/y)=w305:i32)
          n113 = Bundle(cluster=T6 {"Row"=0, "Column"=0} ("Active Cell:Active Cell"), "Row"=w305, "Column"=w304) -> (w307:T6)
          n114 = property on="Grid" class="Tbl (strict)"("Active Cell"=w307, "Cell BG Color"=u32 16777216 ("Active Cell:Cell Background Color")) -> ()  [unwired: 2 in, 2 out]
        }
        n115 = Initialize Array("X", w297, w296) -> (w294:string[][])
        n116 = Bundle By Name(cluster=w299, "Data Acquisition.Partition.Grid"=w294) -> (w295:T1)
        n117 = local write "Grid"(w294) -> ()
        n118 = call <vilib>:"Add State(s) to Queue__JKI_lib_State_Machine.vi"("State(s) in (\"\")"=w301) -> ("States Out"=w302:string)  [unwired: 14 in]
      }
      frame "Grid: Resize" {
        w328 = 21.18 ("y")
        n119 = Unbundle By Name(w327) -> ("Data Acquisition.Partition.Width"=w329:i32, "Data Acquisition.Partition.Height"=w315:i32)
        n120 = case shown="8" w315 {
          tunnel: [i16 870 i16 620] -> w321
          tunnel: [i16 445 ("y") i16 310 ("y")] -> w317
          frame 24, Default {
          }
          frame 8 {
          }
        }
        n121 = Current VI's Path() -> (path=w325:path)
        n122 = Open VI Reference(vi path=w325) -> (vi reference=w326:refnum<vi>, error out=w314:errorcluster)  [unwired: 5 in]
        n123 = property class="VI"(reference=w326, error in=w314) -> (reference out=w324:refnum<vi>, error out=w313:errorcluster, "Front Panel.WinBounds"=w311:T9)
        n124 = Unbundle By Name(w311) -> ("Left"=w322:i16, "Top"=w319:i16)
        n125 = Increment(x=w329) -> (x+1=w332:i32)
        n126 = Increment(x=w315) -> (x+1=w330:i32)
        n127 = Add(x=w322, y=w321) -> (x+y=w320:i16)
        n128 = Add(x=w319, y=w317) -> (x+y=w318:i16)
        n129 = Multiply(x=w332, y=w328) -> (x*y=w333:dbl)
        n130 = Multiply(x=w330, y=w328) -> (x*y=w331:dbl)
        n131 = Bundle By Name(cluster=w311, "Right"=w320, "Bottom"=w318) -> (w323:T9)
        n132 = property on="Grid" class="Tbl (strict)"("Width"=w333, "Height"=w331) -> ()  [unwired: 2 in, 2 out]
        n133 = property class="VI"(reference=w324, error in=w313, "Front Panel.WinBounds"=w323) -> (reference out=w316:refnum<vi>, error out=w312:errorcluster)
        n134 = Close Reference(reference=w316, error in (no error)=w312) -> ()  [unwired: 1 out]
        n135 = call <vilib>:"Add State(s) to Queue__JKI_lib_State_Machine.vi"("State(s) in (\"\")"=w334) -> ("States Out"=w335:string)  [unwired: 14 in]
      }
    }
  }
  "error out" <- w8
  "Canceled?" <- w2
  n136 = case "Cancel?" shown="False" w2 {
    tunnel: [w341 w342] -> w4
    tunnel: w3 -> [w341 _]
    tunnel: "DataCluster in" -> [_ w342]
    frame False {
    }
    frame True {
    }
  }
  "DataCluster out" <- w4
